vi "count down timer.vi"() -> ()   [LabVIEW 2014]
panel:
  out "ms":i32 format="%03d"
  in  "Start / Pause":bool
  out "negitive sign":bool
  in  "second":i32 format="%02d"
  in  "minute":i32 format="%02d"
  in  "hour":i32 format="%02d"
  # "Run the vi and press the start button"
  # "(If the time is negitive, it will be considered to be positive when restarting  )"
  # "(If paused, it will be rounded to 0ms)"
  # "(00:00:00 holds for 3 seconds and then displays the negitive number)"
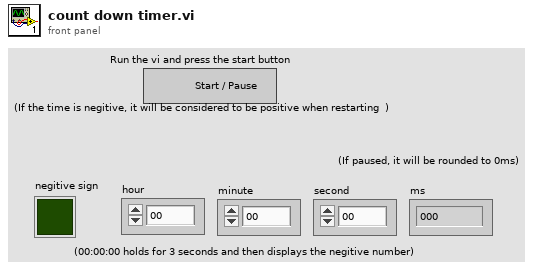
[diagram p1: front panel]
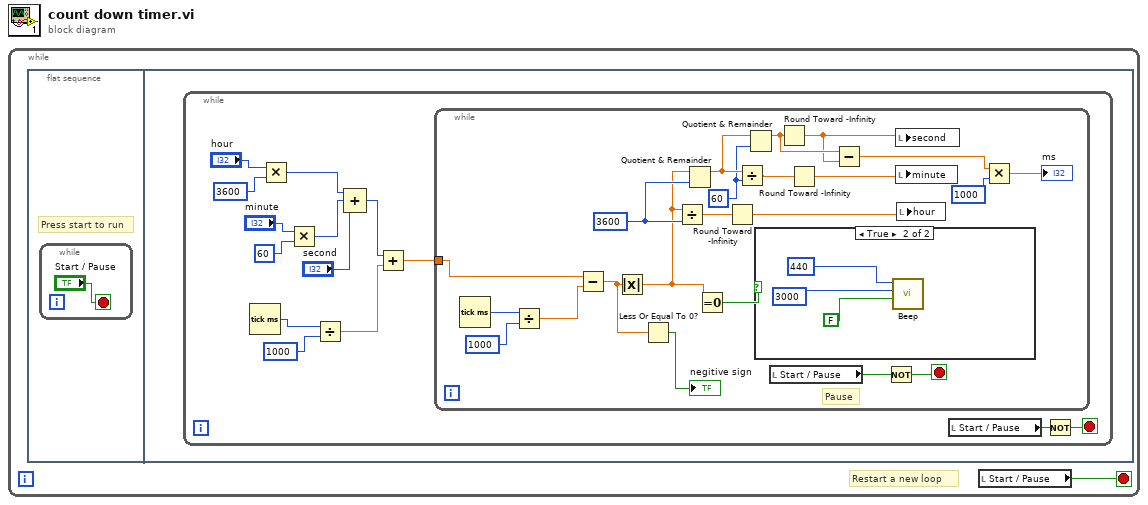
[diagram p0: block diagram]
diagram:
  n1 = while {
    stop <- w1 stop-if-true
    # "Restart a new loop"
    n2 = flat-sequence {
      frame #0 {
        # "Press start to run"
        n3 = while {
          stop <- "Start / Pause" stop-if-true
        }
      }
      frame #1 {
        n4 = while {
          stop <- w4 stop-if-true
          n5 = Tick Count (ms)() -> (millisecond timer value=w10:u32)
          n6 = Multiply(x="hour", y=3600) -> (x*y=w12:i32)
          n7 = Multiply(x="minute", y=60) -> (x*y=w11:i32)
          n8 = Divide(x=w10, y=1000) -> (x/y=w6:dbl)
          n9 = Compound Arithmetic op=ADD(w12, w11, "second") -> (w8:i32)
          n10 = Add(x=w8, y=w6) -> (x+y=w7:dbl)
          n11 = while {
            tunnel: w7 -> [w23]
            stop <- w31 stop-if-true
            w33 = 60
            w35 = 3600
            # "Pause"
            n12 = Tick Count (ms)() -> (millisecond timer value=w37:u32)
            n13 = Divide(x=w37, y=1000) -> (x/y=w30:dbl)
            n14 = Subtract(x=w23, y=w30) -> (x-y=w22:dbl)
            n15 = Absolute Value(x=w22) -> (abs(x)=w27:dbl)
            n16 = Less Or Equal To 0?(x=w22) -> (x <= 0?=→"negitive sign":bool)
            n17 = Divide(x=w27, y=w35) -> (x/y=w28:dbl)
            n18 = Quotient & Remainder(x=w27, y=w35) -> (x-y*floor(x/y)=w34:dbl)  [unwired: 1 out]
            n19 = Equal To 0?(x=w27) -> (x = 0?=w29:bool)
            n20 = Round Toward -Infinity(1:w28) -> (0:w26:dbl)
            n21 = Divide(x=w34, y=w33) -> (x/y=w25:dbl)
            n22 = Quotient & Remainder(x=w34, y=w33) -> (x-y*floor(x/y)=w21:dbl)  [unwired: 1 out]
            n23 = case shown="True" w29 {
              frame False {
              }
              frame True {
                n24 = call <vilib>:"Beep.vi"("use system alert? (T)"=FALSE, "duration (msec)"=u32 3000, "frequency (Hz)"=u32 440) -> ()  [unwired: 9 in]
              }
            }
            n25 = local read "Start / Pause"() -> (w32:bool)
            n26 = Round Toward -Infinity(1:w21) -> (0:w20:dbl)
            n27 = Round Toward -Infinity(1:w25) -> (0:w24:dbl)
            n28 = Subtract(x=w21, y=w20) -> (x-y=w19:dbl)
            n29 = Not(x=w32) -> (.not. x?=w31:bool)
            n30 = local write "second"(w20) -> ()
            n31 = local write "minute"(w24) -> ()
            n32 = local write "hour"(w26) -> ()
            n33 = Multiply(x=w19, y=1000) -> (x*y=→"ms":dbl)
          }
          n34 = local read "Start / Pause"() -> (w5:bool)
          n35 = Not(x=w5) -> (.not. x?=w4:bool)
        }
      }
    }
    n36 = local read "Start / Pause"() -> (w1:bool)
  }
